vi "ActiveX Child Window.vi"() -> ()   [LabVIEW 2016]
uses:
  USER32.DLL
panel:
  in  "WebBrowser":refnum<k7>(container)
  out "hWnd 3":u32
  out "error out":errorcluster
  out "hWnd 2":u32
  out "hWnd":u32
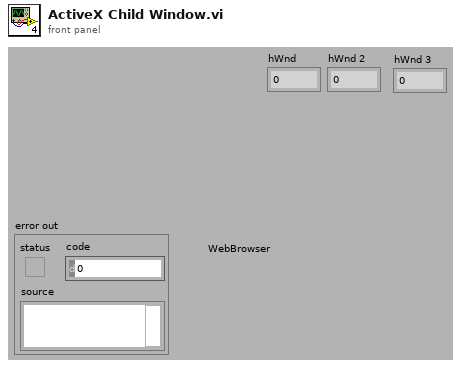
[diagram p1: front panel]
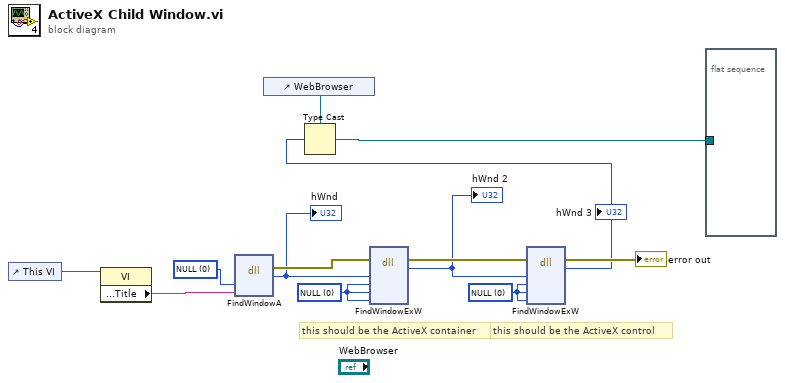
[diagram p0: block diagram]
diagram:
  w7 = 0 items=["NULL"]
  w10 = 0 items=["NULL"]
  w13 = 0 items=["NULL"]
  # "this should be the ActiveX control"
  # "this should be the ActiveX container"
  n1 = control-ref of="This VI"() -> (w12:refnum<vi>)
  n2 = property class="VI"(reference=w12) -> ("Front Panel Window:Title"=w11:string)  [unwired: 1 in, 2 out]
  n3 = dll-call lib="user32.dll" fn="FindWindowA" label="FindWindow"("lpszClassName"=w13, "lpszWindowName"=w11) -> (error out=w9:errorcluster, "hWnd"=w3:u32)  [unwired: 5 in, 1 out]
  "hWnd" <- w3
  n4 = control-ref of="WebBrowser"() -> (w4:refnum<vi>)
  n5 = dll-call lib="user32.dll" fn="FindWindowExW" label="FindWindowEx"(error in=w9, "hwndParent"=w3, "hwndChildAfter"=w10, "lpszClassName"=w10, "lpszWindowName"=w10) -> (error out=w8:errorcluster, "hWnd"=w2:u32)  [unwired: 6 in, 1 out]
  "hWnd 2" <- w2
  n6 = dll-call lib="user32.dll" fn="FindWindowExW" label="FindWindowEx"(error in=w8, "hwndParent"=w2, "hwndChildAfter"=w7, "lpszClassName"=w7, "lpszWindowName"=w7) -> (error out=→"error out":errorcluster, "hWnd"=w1:u32)  [unwired: 6 in, 1 out]
  "hWnd 3" <- w1
  n7 = Type Cast(type=w4, x=w1) -> (*(type *) &x=w5:refnum<vi>)
  n8 = flat-sequence {
    tunnel: w5 -> [_]
    frame #0 {
    }
  }
